vi "Pot Line.vi"(8 "error in":errorcluster, 9 "End Position":refnum<class "Vec3d Class.lvclass">, 10 "Start Position":refnum<class "Vec3d Class.lvclass">, 11 "SyringeTool in":refnum<class "SyringeTool Class.lvclass">) -> (0 "error out":errorcluster, 3 "SyringeTool out":refnum<class "SyringeTool Class.lvclass">)   [LabVIEW 2011, in "SyringeTool Class.lvclass"]
uses:
  SyringeTool Class.lvclass
  Vec3d Class/Vec3d Class.lvclass
  WorkTable Class/WorkTable Class.lvclass
  Config Manager Class/Config Manager Class.lvclass
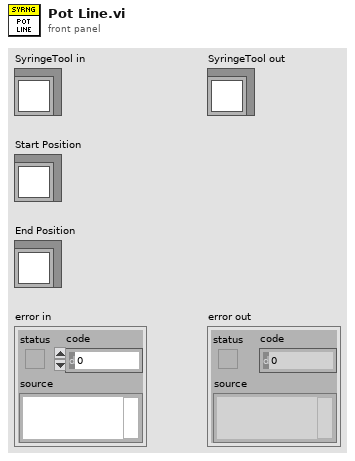
[diagram p1: front panel]
types:
  T1 = typedef "Potting Parameters.ctl" = cluster{"Curing Param A":dbl, "Curing Param B":dbl, "Speed Nominal":dbl, "Time Nominal":dbl, "Turn-on Time":dbl, "Turn-off Time":dbl, "Safe Height Offset":dbl, "Tip Height":dbl}
  T2 = typedef "Worktable_Syringe.ctl" = cluster{"Syringe Holder":enum16{"Empty", "Populated", "Calibrated"}, "Mixing Time":timestamp, "Tip Offset":refnum<class "Vec3d Class.lvclass">}
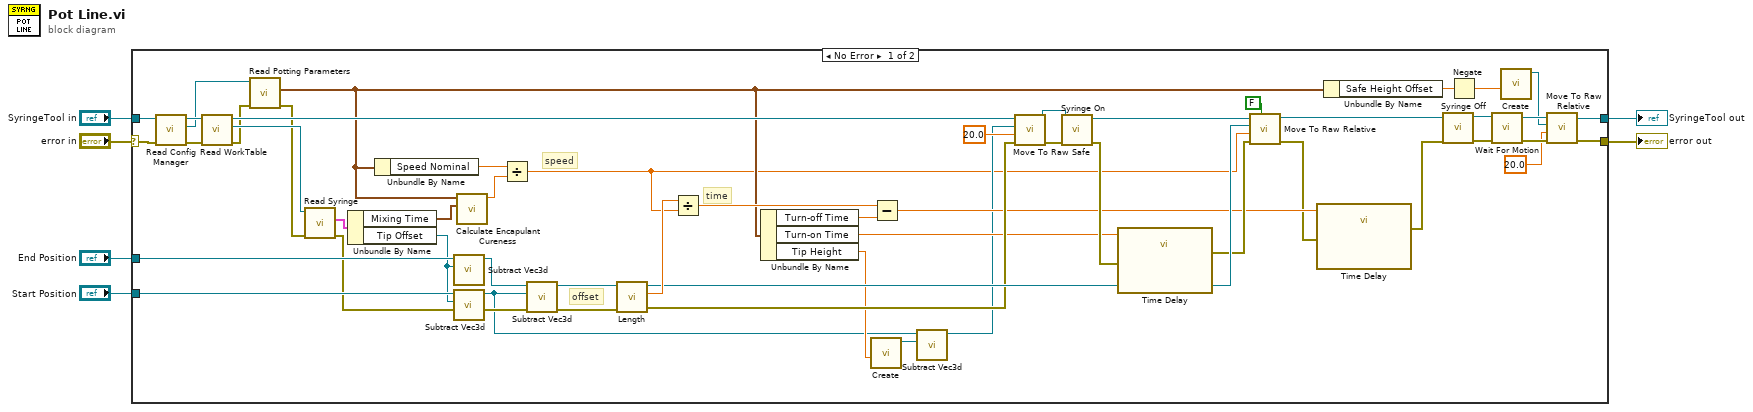
[diagram p0: block diagram]
diagram:
  n1 = case shown="No Error" "error in" {
    selector: "error in" -> [w19 w61]
    tunnel: [w46 w61] -> w5
    tunnel: [w51 w60] -> w3
    tunnel: "SyringeTool in" -> [w29 w60]
    tunnel: "Start Position" -> [w44 _]
    tunnel: "End Position" -> [w42 _]
    frame No Error {
      # "offset"
      # "speed"
      # "time"
      n2 = call-dynamic "Read Config Manager.vi"("error in"=w19, "Gantry in"=w29) -> ("error out"=w22:errorcluster, "Config Manager"=w23:refnum<class "Config Manager Class.lvclass">, "Gantry out"=w28:refnum<class "SyringeTool Class.lvclass">)  [unwired: 7 in]
      n3 = call-dynamic "Read WorkTable.vi"("error in"=w22, "Gantry Class in"=w28) -> ("error out"=w21:errorcluster, "WorkTable Class.lvclass"=w59:refnum<class "WorkTable Class.lvclass">, "Gantry Class out"=w43:refnum<class "SyringeTool Class.lvclass">)  [unwired: 7 in]
      n4 = call "Read Potting Parameters.vi"("error in"=w21, "Config Manager in"=w23) -> ("error out"=w20:errorcluster, "Potting Parameters"=w10:T1)  [unwired: 7 in, 1 out]
      n5 = call "Read Syringe.vi"("error in"=w20, "WorkTable in"=w59) -> ("error out"=w18:errorcluster, "Syringe"=w58:T2)  [unwired: 7 in, 1 out]
      n6 = Unbundle By Name(w58) -> ("Mixing Time"=w11:timestamp, "Tip Offset"=w41:refnum<class "Vec3d Class.lvclass">)
      n7 = Unbundle By Name(w10) -> ("Speed Nominal"=w9:dbl)
      n8 = call "Subtract Vec3d.vi"("Vec3d in 2"=w41, "Vec3d in 1"=w42) -> ("Vec3d Class out"=w45:refnum<class "Vec3d Class.lvclass">)  [unwired: 8 in, 1 out]
      n9 = call "Subtract Vec3d.vi"("Vec3d in 2"=w41, "Vec3d in 1"=w44) -> ("Vec3d Class out"=w14:refnum<class "Vec3d Class.lvclass">)  [unwired: 8 in, 1 out]
      n10 = call "Calculate Encapulant Cureness.vi"("Mixing Time"=w11, "Potting Parameters"=w10) -> ("Cureness"=w8:dbl)  [unwired: 9 in]
      n11 = Divide(x=w9, y=w8) -> (x/y=w7:dbl)
      n12 = call "Subtract Vec3d.vi"("error in (no error)"=w18, "Vec3d in 2"=w14, "Vec3d in 1"=w45) -> ("error out"=w40:errorcluster, "Vec3d Class out"=w56:refnum<class "Vec3d Class.lvclass">)  [unwired: 7 in]
      n13 = call-dynamic "Length.vi"("error in"=w40, "Vec3d in"=w56) -> ("error out"=w39:errorcluster, "Length"=w57:dbl, "Vec3d out"=w55:refnum<class "Vec3d Class.lvclass">)  [unwired: 7 in]
      n14 = Divide(x=w57, y=w7) -> (x/y=w54:dbl)
      n15 = Unbundle By Name(w10) -> ("Turn-off Time"=w25:dbl, "Turn-on Time"=w24:dbl, "Tip Height"=w15:dbl)
      n16 = call "Create.vi"("Z"=w15) -> ("Vec3d Class out"=w12:refnum<class "Vec3d Class.lvclass">)  [unwired: 9 in, 1 out]
      n17 = Subtract(x=w54, y=w25) -> (x-y=w35:dbl)
      n18 = call "Subtract Vec3d.vi"("Vec3d in 2"=w12, "Vec3d in 1"=w14) -> ("Vec3d Class out"=w13:refnum<class "Vec3d Class.lvclass">)  [unwired: 8 in, 1 out]
      n19 = call-dynamic "Move To Raw Safe.vi"("error in"=w39, "Speed(mm/s)"=20.0, "Destination"=w13, "Gantry in"=w43) -> ("error out"=w37:errorcluster, "Gantry out"=w36:refnum<class "SyringeTool Class.lvclass">)  [unwired: 6 in]
      n20 = call "Syringe On.vi"("error in"=w37, "SyringeTool"=w36) -> ("error out"=w38:errorcluster, "SyringeTool out"=w53:refnum<class "SyringeTool Class.lvclass">)  [unwired: 8 in]
      n21 = call "Time Delay"("error in (no error)"=w38, "Delay Time (s)"=w24) -> ("error out"=w49:errorcluster)  [unwired: 9 in]
      n22 = call-dynamic "Move To Raw Relative.vi"("Wait?"=FALSE, "error in"=w49, "Speed(mm/s)"=w7, "Delta"=w55, "Gantry in"=w53) -> ("error out"=w33:errorcluster, "Gantry out"=w52:refnum<class "SyringeTool Class.lvclass">)  [unwired: 5 in]
      n23 = call "Time Delay"("error in (no error)"=w33, "Delay Time (s)"=w35) -> ("error out"=w48:errorcluster)  [unwired: 9 in]
      n24 = Unbundle By Name(w10) -> ("Safe Height Offset"=w27:dbl)
      n25 = call "Syringe Off.vi"("error in"=w48, "SyringeTool in"=w52) -> ("error out"=w32:errorcluster, "SyringeTool out"=w31:refnum<class "SyringeTool Class.lvclass">)  [unwired: 8 in]
      n26 = Negate(x=w27) -> (-x=w26:dbl)
      n27 = call-dynamic "Wait For Motion.vi"("error in"=w32, "Gantry in"=w31) -> ("error out"=w47:errorcluster, "Gantry out"=w50:refnum<class "SyringeTool Class.lvclass">)  [unwired: 8 in]
      n28 = call "Create.vi"("Z"=w26) -> ("Vec3d Class out"=w30:refnum<class "Vec3d Class.lvclass">)  [unwired: 9 in, 1 out]
      n29 = call-dynamic "Move To Raw Relative.vi"("error in"=w47, "Speed(mm/s)"=20.0, "Delta"=w30, "Gantry in"=w50) -> ("error out"=w46:errorcluster, "Gantry out"=w51:refnum<class "SyringeTool Class.lvclass">)  [unwired: 6 in]
    }
    frame Error {
    }
  }
  "error out" <- w5
  "SyringeTool out" <- w3
